vi "GetWIPDataWithM100.vi"(8 "error in":errorcluster, 10 "Lotno":string="A141100029", 11 "connection reference":T1) -> (0 "error out":errorcluster, 1 "output array":string[][](array[string]), 2 "data":i32, 3 "connection reference 2":T1)   [LabVIEW 2012]
uses:
  <vilib>/addons/database/Connection.llb/Conn ObjectReference.ctl
  <vilib>/addons/database/Auxilliary.llb/DB Tools Cursor Type.ctl
  <vilib>/addons/database/Connection.llb/Conn Execute.vi
  <vilib>/addons/database/Recordset.llb/Rec Fetch Integer Data (R).vi
  <vilib>/addons/database/Recordset.llb/Rec Destroy - Connection.vi
  <vilib>/addons/database/Recordset.llb/Rec Fetch Recordset Data (R).vi
  <vilib>/addons/database/_DB Variant To Data/Database Variant To Data.xnode
  <vilib>/addons/database/NI_Database_API.lvlib
panel:
  out "concatenated string":string
  out "error out 2":errorcluster
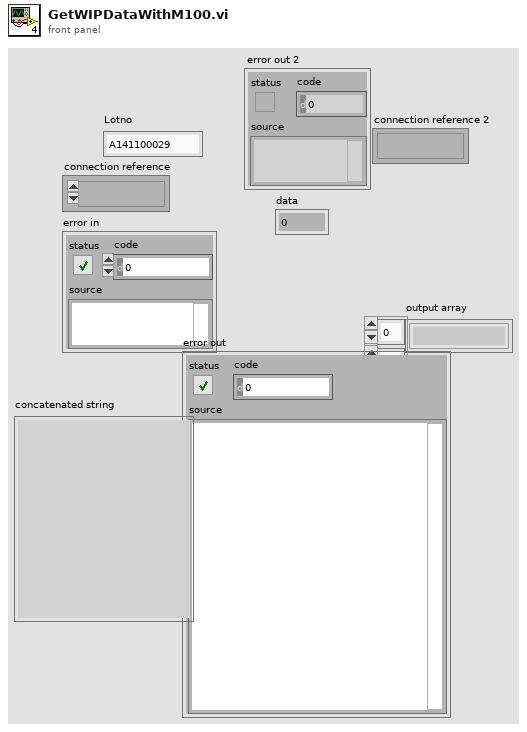
[diagram p1: front panel]
types:
  T1 = typedef "NI_Database_API.lvlib/Conn ObjectReference.ctl" = refnum<k1>
  T2 = typedef "NI_Database_API.lvlib/DB Tools Cursor Type.ctl" = enum16{"forward-only", "keyset", "dynamic", "static"}
  T3 = typedef "NI_Database_API.lvlib/Rec ObjectReference.ctl" = refnum<k1>
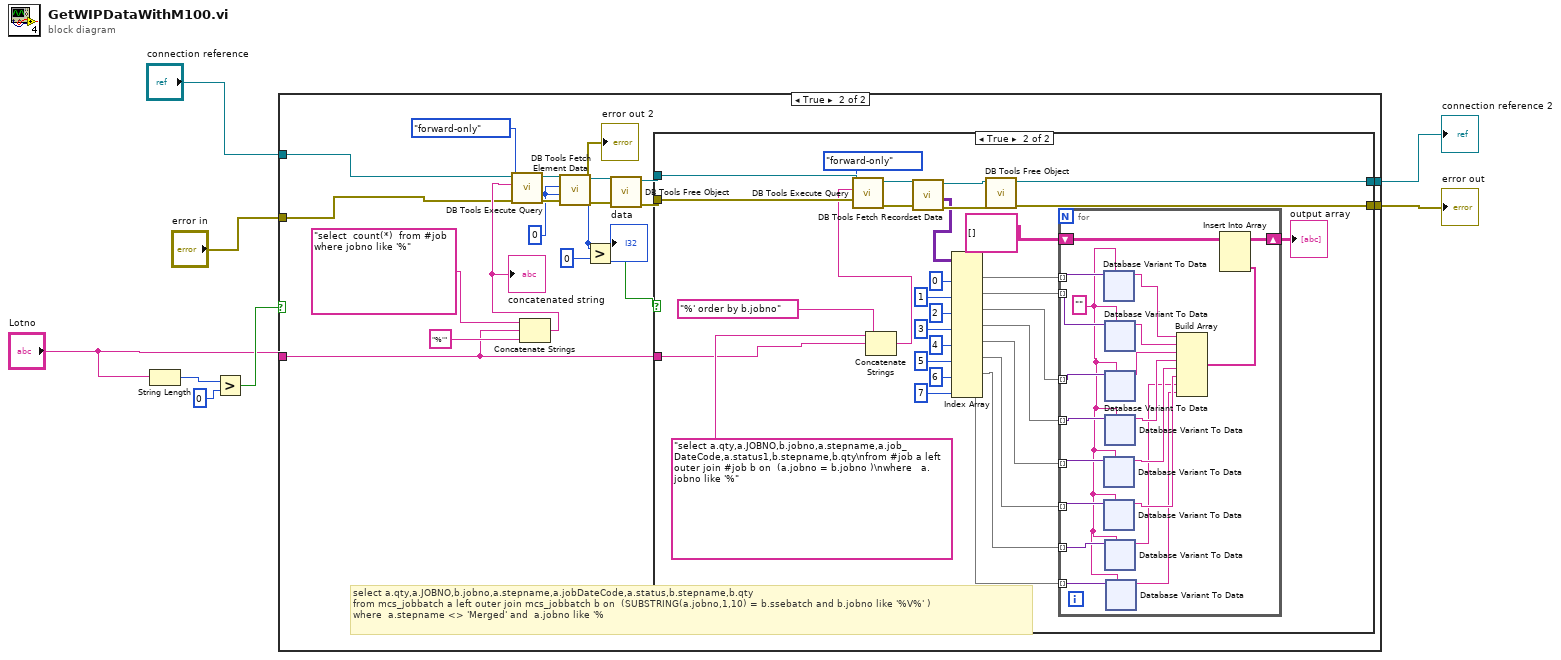
[diagram p0: block diagram]
diagram:
  n1 = String Length(string="Lotno") -> (length=w8:i32)
  n2 = Greater?(x=w8, y=0) -> (0:w6:bool)
  n3 = case shown="True" w6 {
    tunnel: "Lotno" -> [_ w25]
    tunnel: "error in" -> [w9 w14]
    tunnel: "connection reference" -> [w10 w13]
    tunnel: [w10 w12] -> w2
    tunnel: [w9 w11] -> w1
    frame False {
    }
    frame True {
      w18 = 0
      # "select a.qty,a.JOBNO,b.jobno,a.stepname,a.jobDateCode,a.status,b.stepname,b.qty\nfrom mcs_jobbatch a left outer join mcs_jobbatch b on  (SUBSTRING(a.jobno,1,10) = b.ssebatch and b.jobno like '%V%' )\nwhere  a.stepname <> 'Merged' and  a.jobno like '%"
      n4 = Concatenate Strings("select  count(*)  from #job where jobno like '%" ("string"), w25, "%'" ("string")) -> (w23:string)
      "concatenated string" <- w23
      n5 = call-poly <vilib>:"DB Tools Execute Query.vi"("error in (no error)"=w14, "cursor type"=DB_Tools_Cursor_Type."forward-only", "SQL query"=w23, "connection reference"=w13) -> ("error out"=w22:errorcluster, "recordset reference"=w21:T3)  [unwired: 4 in]
      n6 = call-poly <vilib>:"DB Tools Fetch Element Data.vi"("error in (no error)"=w22, "type"=w18, "column index"=w18, "recordset reference"=w21) -> ("error out"=w19:errorcluster, "data"=w17:i32, "recordset reference out"=w20:T3)  [unwired: 3 in]
      "data" <- w17
      "error out 2" <- w19
      n7 = Greater?(x=w17, y=0) -> (0:w15:bool)
      n8 = call-poly <vilib>:"DB Tools Free Object.vi"("error in (no error)"=w19, "recordset reference"=w20) -> ("error out"=w28:errorcluster, "connection reference"=w29:T1)  [unwired: 8 in]
      n9 = case shown="True" w15 {
        tunnel: w29 -> [w31 w63]
        tunnel: w28 -> [w30 w60]
        tunnel: w25 -> [_ w53]
        tunnel: [w31 w52] -> w12
        tunnel: [w30 w51] -> w11
        frame False {
        }
        frame True {
          n10 = Concatenate Strings("select a.qty,a.JOBNO,b.jobno,a.stepname,a.job_DateCode,a.status1,b.stepname,b.qty\nfrom #job a left outer join #job b on  (a.jobno = b.jobno )\nwhere   a.jobno like '%" ("string"), w53, "%' order by b.jobno" ("string")) -> (w54:string)
          n11 = call-poly <vilib>:"DB Tools Execute Query.vi"("error in (no error)"=w60, "cursor type"=DB_Tools_Cursor_Type."forward-only", "SQL query"=w54, "connection reference"=w63) -> ("error out"=w59:errorcluster, "recordset reference"=w62:T3)  [unwired: 4 in]
          n12 = call-poly <vilib>:"DB Tools Fetch Recordset Data.vi"("error in (no error)"=w59, "recordset reference"=w62) -> ("error out"=w58:errorcluster, "recordset data"=w50:variant[][], "recordset reference out"=w61:T3)  [unwired: 3 in]
          n13 = Index Array(array=w50, index (col) #1=0 ("disabled index (col)"), index (col) #2=1 ("index (col)"), index (col) #3=2 ("index (col)"), index (col) #4=3 ("index (col)"), index (col) #5=4 ("index (col)"), index (col) #6=5 ("index (col)"), index (col) #7=6 ("index (col)"), index (col) #8=7 ("index (col)")) -> (element #1=w43:variant[], element #2=w42:variant[], element #3=w41:variant[], element #4=w40:variant[], element #5=w39:variant[], element #6=w38:variant[], element #7=w33:variant[], element #8=w32:variant[])  [unwired: 8 in]
          n14 = call-poly <vilib>:"DB Tools Free Object.vi"("error in (no error)"=w58, "recordset reference"=w61) -> ("error out"=w51:errorcluster, "connection reference"=w52:T1)  [unwired: 8 in]
          n15 = for {
            tunnel: w43 -> [w83] mode=indexing
            tunnel: w42 -> [w82] mode=indexing
            tunnel: w41 -> [w81] mode=indexing
            tunnel: w40 -> [w80] mode=indexing
            tunnel: w39 -> [w79] mode=indexing
            tunnel: w38 -> [w78] mode=indexing
            shift-right: [w70] -> w36
            shift-left: string[][] [] ("output array") -> [w69]
            tunnel: w33 -> [w68] mode=indexing
            tunnel: w32 -> [w66] mode=indexing
            w65 = ""
            n16 = xnode "Database Variant To Data"("database variant"=w83, "type"=w65) -> ("data"=w77:string)  [unwired: 1 in, 1 out]
            n17 = xnode "Database Variant To Data"("database variant"=w79, "type"=w65) -> ("data"=w73:string)  [unwired: 1 in, 1 out]
            n18 = xnode "Database Variant To Data"("database variant"=w78, "type"=w65) -> ("data"=w72:string)  [unwired: 1 in, 1 out]
            n19 = xnode "Database Variant To Data"("database variant"=w82, "type"=w65) -> ("data"=w76:string)  [unwired: 1 in, 1 out]
            n20 = xnode "Database Variant To Data"("database variant"=w81, "type"=w65) -> ("data"=w75:string)  [unwired: 1 in, 1 out]
            n21 = xnode "Database Variant To Data"("database variant"=w80, "type"=w65) -> ("data"=w74:string)  [unwired: 1 in, 1 out]
            n22 = xnode "Database Variant To Data"("database variant"=w68, "type"=w65) -> ("data"=w67:string)  [unwired: 1 in, 1 out]
            n23 = xnode "Database Variant To Data"("database variant"=w66, "type"=w65) -> ("data"=w64:string)  [unwired: 1 in, 1 out]
            n24 = Build Array(w77, w76, w75, w74, w73, w72, w67, w64) -> (w71:string[])
            n25 = Insert Into Array(array=w69, new element=w71) -> (w70:string[][])  [unwired: 2 in]
          }
          "output array" <- w36
        }
      }
    }
  }
  "connection reference 2" <- w2
  "error out" <- w1
